vi "sound_play.vi"() -> ()   [LabVIEW 2015]
panel:
  out "is playing?":bool
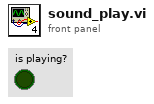
[diagram p1: front panel]
types:
  T1 = typedef "Sound Output Task ID.ctl" = u32
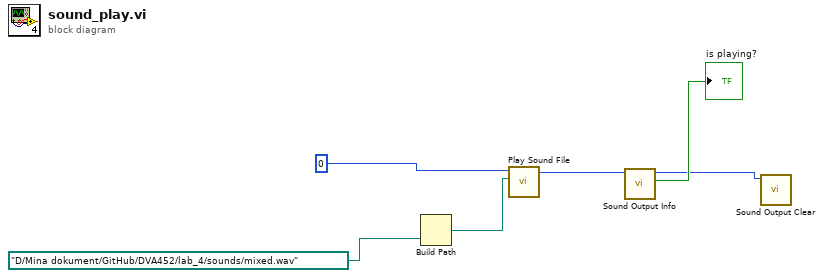
[diagram p0: block diagram]
diagram:
  n1 = Build Path(name or relative path=path "D:/Mina dokument/GitHub/DVA452/lab_4/sounds/mixed.wav" ("base path")) -> (appended path=w2:path)  [unwired: 1 in]
  n2 = call <vilib>:"Play Sound File.vi"("path"=w2, "device ID"=u32 0) -> ("task ID"=w1:T1)  [unwired: 8 in, 1 out]
  n3 = call <vilib>:"Sound Output Info.vi"("task ID"=w1) -> ("is playing?"=→"is playing?":bool, "task ID out"=w3:T1)  [unwired: 7 in, 2 out]
  n4 = call <vilib>:"Sound Output Clear.vi"("task ID"=w3) -> ()  [unwired: 10 in, 1 out]
